vi "S2DS_DetermineTargetInX.vi"(2 "Measurement ON?":bool, 3 "Scan parameters  in":T1 {"Y data taking" items=["in both direction", "in up direction only", "in down direction only"]; "X data taking" items=["in both direction", "in up direction only", "in down direction only"]}) -> (0 "Change  x direction":bool, 1 "Scan parameters  out":T1 {"Y data taking" items=["in both direction", "in up direction only", "in down direction only"]; "X data taking" items=["in both direction", "in up direction only", "in down direction only"]})   [LabVIEW 2025]
uses:
  TYPE DEFS/S2DS_Sweep Info.ctl
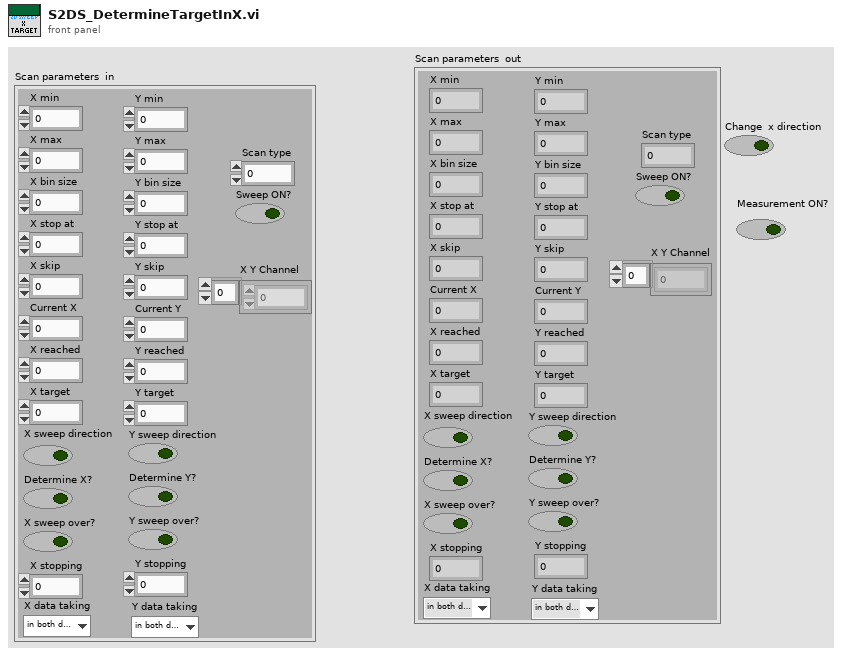
[diagram p1: front panel]
types:
  T1 = typedef "S2DS_Sweep Info.ctl" = cluster{"X min":ext, "X max":dbl, "Y min":dbl, "Y max":dbl, "X bin size":dbl, "Y bin size":dbl, "X stop at":dbl, "Y stop at":dbl, "X skip":u64, "Y skip":u64, "Current X":dbl, "Current Y":dbl, "X reached":i32, "Y reached":i32, "X target":dbl, "Y target":dbl, "Sweep ON?":bool, "X sweep direction":bool, "Y sweep direction":bool, "Determine X?":bool, "Determine Y?":bool, "X sweep over?":bool, "Y sweep over?":bool, "Scan type":i32, "X stopping":i32, "Y stopping":i32, "X Y Channel":u16[], "X data taking":u16, "Y data taking":u16}
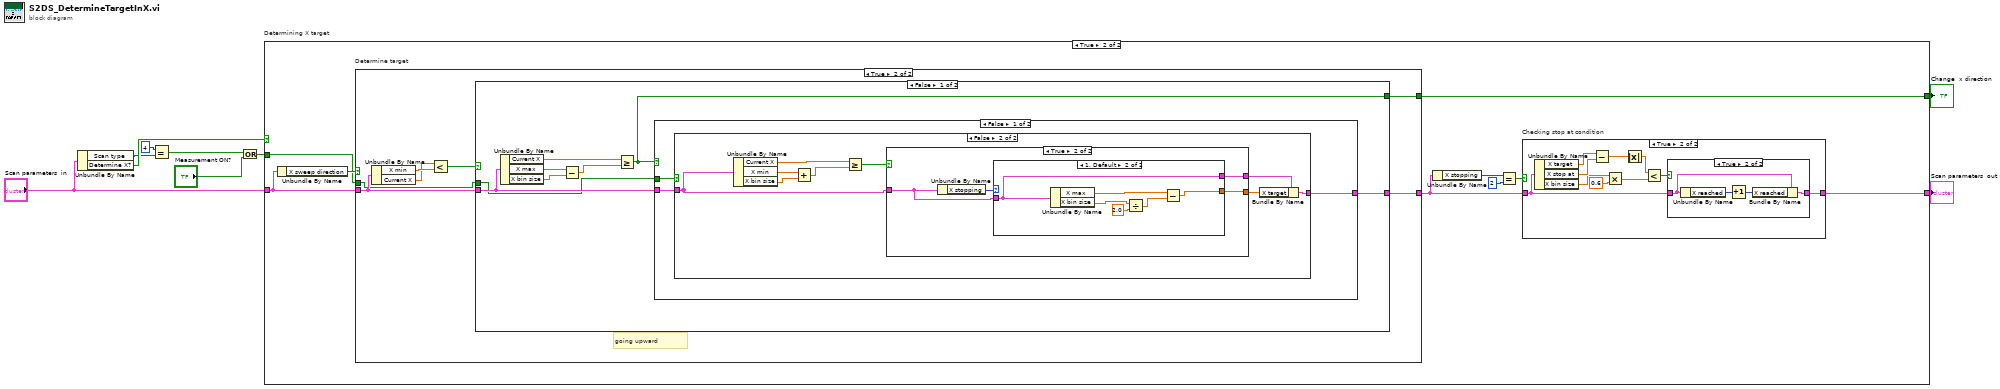
[diagram p0: block diagram]
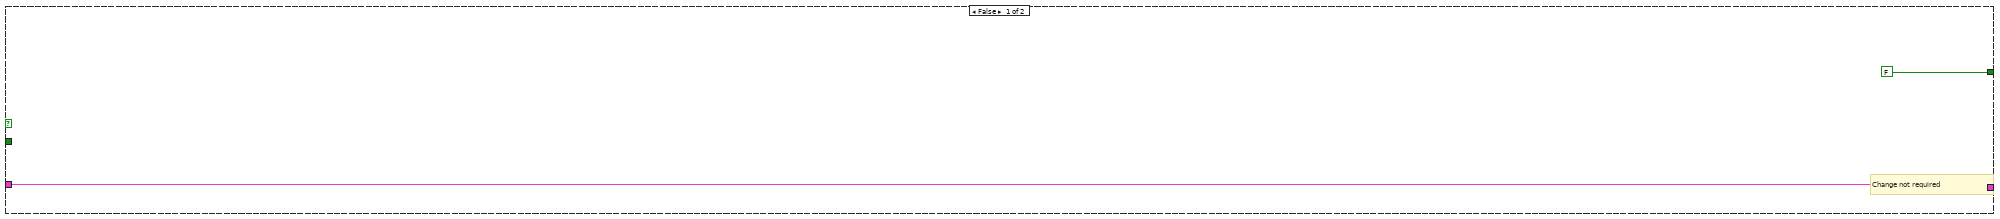
[diagram p2: hidden frame]
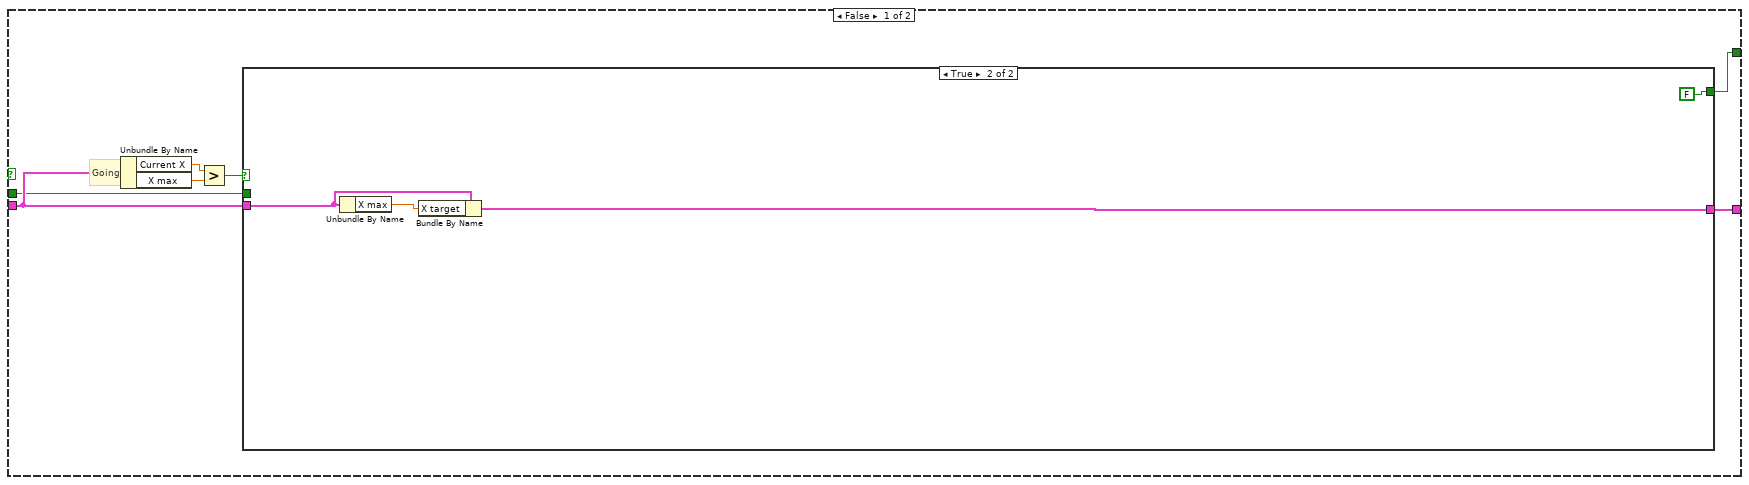
[diagram p3: hidden frame]
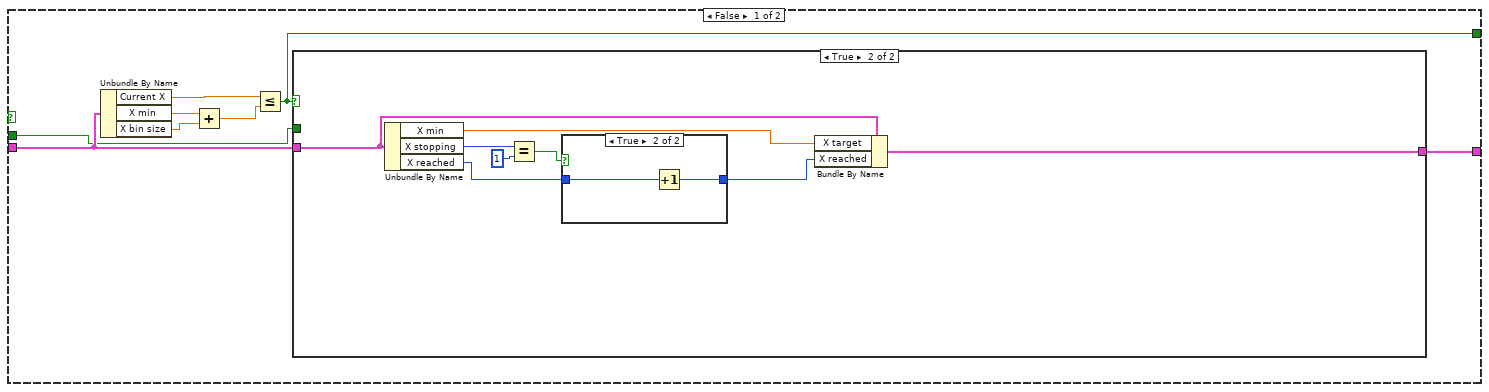
[diagram p4: hidden frame]
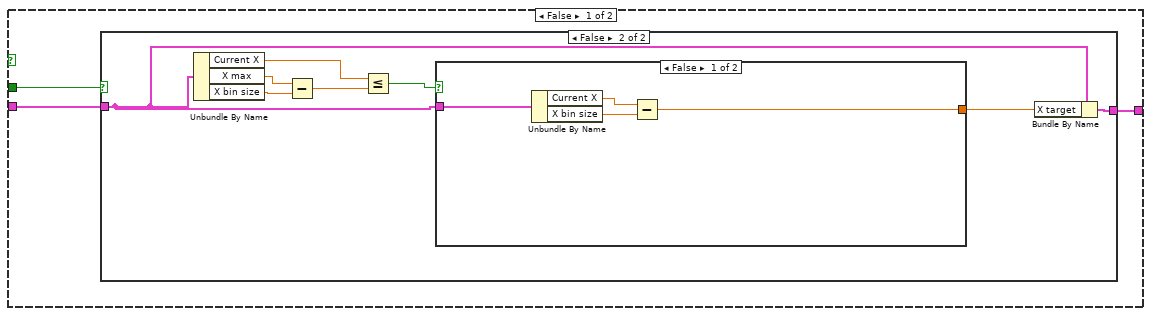
[diagram p5: hidden frame]
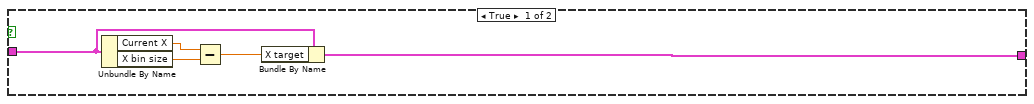
[diagram p6: hidden frame]
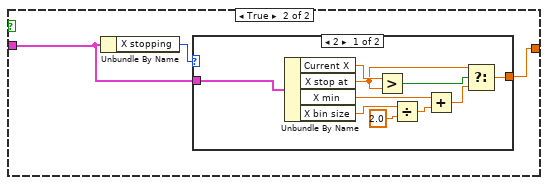
[diagram p7: hidden frame]
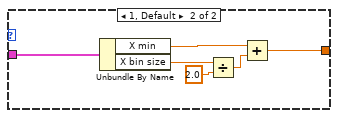
[diagram p8: hidden frame]
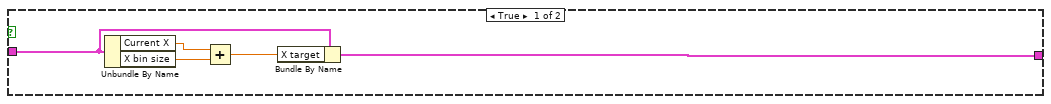
[diagram p10: hidden frame]
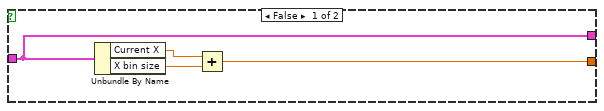
[diagram p11: hidden frame]
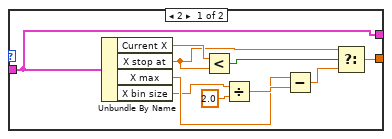
[diagram p12: hidden frame]
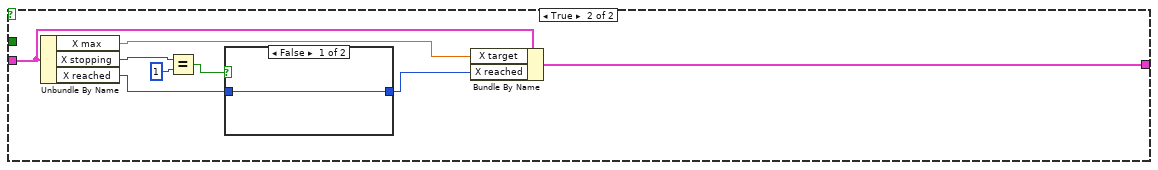
[diagram p13: hidden frame]
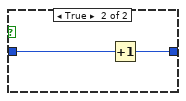
[diagram p14: hidden frame]
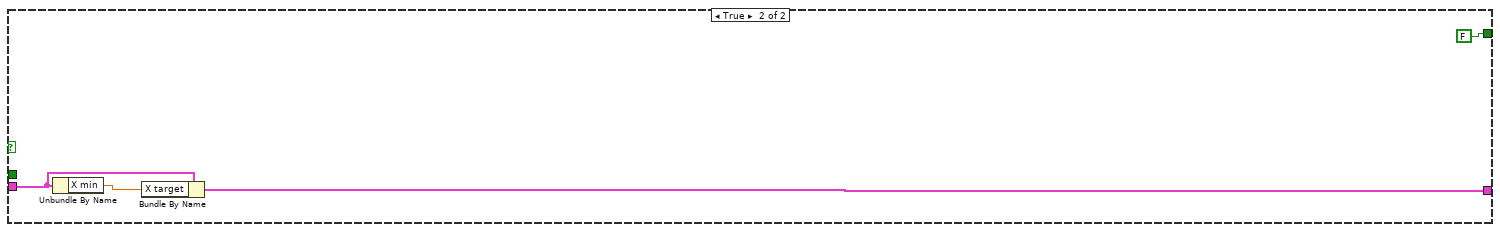
[diagram p15: hidden frame]
diagram:
  n1 = Unbundle By Name("Scan parameters  in") -> ("Scan type"=w5:i32, "Determine X?"=w7:bool)
  n2 = Equal?(x=4, y=w5) -> (x = y?=w3:bool)
  n3 = Or(x=w3, y="Measurement ON?") -> (x .or. y?=w1:bool)
  n4 = case "Determining X target" shown="True" w7 {
    tunnel: "Scan parameters  in" -> [w11 w20]
    tunnel: [w11 w14] -> w9
    tunnel: [FALSE w13] -> w6
    tunnel: w1 -> [_ w12]
    frame False {
      # "Change not required"
    }
    frame True {
      n5 = Unbundle By Name(w20) -> ("X sweep direction"=w18:bool)
      n6 = case "Determine target" shown="True" w18 {
        tunnel: w20 -> [w27 w93]
        tunnel: [w26 w92] -> w19
        tunnel: [w22 w91] -> w13
        tunnel: w12 -> [w21 w90]
        frame False {
          # "Going down"
          n7 = Unbundle By Name(w27) -> ("Current X"=w25:dbl, "X max"=w24:dbl)
          n8 = Greater?(x=w25, y=w24) -> (0:w23:bool)
          n9 = case shown="True" w23 {
            tunnel: w27 -> [w31 w89]
            tunnel: [w30 w87] -> w26
            tunnel: [w29 FALSE] -> w22
            tunnel: w21 -> [w28 _]
            frame False {
              n10 = Unbundle By Name(w31) -> ("Current X"=w33:dbl, "X min"=w35:ext, "X bin size"=w34:dbl)
              n11 = Add(x=w35, y=w34) -> (x+y=w32:ext)
              n12 = Less Or Equal?(x=w33, y=w32) -> (x <= y?=w29:bool)
              n13 = case shown="True" w29 {
                tunnel: w31 -> [w38 w82]
                tunnel: [w37 w80] -> w30
                tunnel: w28 -> [w36 _]
                frame False {
                  n14 = case shown="False" w36 {
                    tunnel: w38 -> [w43 w49]
                    tunnel: [w42 w51] -> w37
                    frame True {
                      n15 = Unbundle By Name(w43) -> ("Current X"=w41:dbl, "X bin size"=w40:dbl)
                      n16 = Subtract(x=w41, y=w40) -> (x-y=w39:dbl)
                      n17 = Bundle By Name(cluster=w43, "X target"=w39) -> (w42:T1)
                    }
                    frame False {
                      n18 = Unbundle By Name(w49) -> ("Current X"=w46:dbl, "X max"=w48:dbl, "X bin size"=w47:dbl)
                      n19 = Subtract(x=w48, y=w47) -> (x-y=w45:dbl)
                      n20 = Less Or Equal?(x=w46, y=w45) -> (x <= y?=w44:bool)
                      n21 = case shown="False" w44 {
                        tunnel: [w52 w58] -> w50
                        tunnel: w49 -> [w53 w57]
                        frame False {
                          n22 = Unbundle By Name(w53) -> ("Current X"=w55:dbl, "X bin size"=w54:dbl)
                          n23 = Subtract(x=w55, y=w54) -> (x-y=w52:dbl)
                        }
                        frame True {
                          n24 = Unbundle By Name(w57) -> ("X stopping"=w56:i32)
                          n25 = case shown="2" w56 {
                            tunnel: w57 -> [w68 w74]
                            tunnel: [w64 w72] -> w58
                            frame 2 {
                              n26 = Unbundle By Name(w68) -> ("Current X"=w67:dbl, "X stop at"=w65:dbl, "X min"=w63:ext, "X bin size"=w62:dbl)
                              n27 = Greater?(x=w67, y=w65) -> (0:w66:bool)
                              n28 = Divide(x=w62, y=2.0) -> (x/y=w60:dbl)
                              n29 = Add(x=w63, y=w60) -> (x+y=w59:ext)
                              n30 = Select(t=w65, s=w66, f=w59) -> (s? t:f=w64:ext)
                            }
                            frame 1, Default {
                              n31 = Unbundle By Name(w74) -> ("X min"=w73:ext, "X bin size"=w71:dbl)
                              n32 = Divide(x=w71, y=2.0) -> (x/y=w69:dbl)
                              n33 = Add(x=w73, y=w69) -> (x+y=w72:ext)
                            }
                          }
                        }
                      }
                      n34 = Bundle By Name(cluster=w49, "X target"=w50) -> (w51:T1)
                    }
                  }
                }
                frame True {
                  n35 = Unbundle By Name(w82) -> ("X min"=w81:ext, "X stopping"=w75:i32, "X reached"=w79:i32)
                  n36 = Equal?(x=w75, y=1) -> (x = y?=w76:bool)
                  n37 = case shown="True" w76 {
                    tunnel: w79 -> [w83 w85]
                    tunnel: [w83 w84] -> w78
                    frame False {
                    }
                    frame True {
                      n38 = Increment(x=w85) -> (x+1=w84:i32)
                    }
                  }
                  n39 = Bundle By Name(cluster=w82, "X target"=w81, "X reached"=w78) -> (w80:T1)
                }
              }
            }
            frame True {
              n40 = Unbundle By Name(w89) -> ("X max"=w88:dbl)
              n41 = Bundle By Name(cluster=w89, "X target"=w88) -> (w87:T1)
            }
          }
        }
        frame True {
          # "going upward"
          n42 = Unbundle By Name(w93) -> ("X min"=w96:ext, "Current X"=w95:dbl)
          n43 = Less?(x=w95, y=w96) -> (x < y?=w94:bool)
          n44 = case shown="False" w94 {
            tunnel: w93 -> [w100 w160]
            tunnel: [w99 w158] -> w92
            tunnel: [w98 FALSE] -> w91
            tunnel: w90 -> [w97 _]
            frame False {
              n45 = Unbundle By Name(w100) -> ("Current X"=w102:dbl, "X max"=w104:dbl, "X bin size"=w103:dbl)
              n46 = Subtract(x=w104, y=w103) -> (x-y=w101:dbl)
              n47 = Greater Or Equal?(x=w102, y=w101) -> (x >= y?=w98:bool)
              n48 = case shown="False" w98 {
                tunnel: w100 -> [w107 w153]
                tunnel: [w106 w151] -> w99
                tunnel: w97 -> [w105 _]
                frame False {
                  n49 = case shown="False" w105 {
                    tunnel: w107 -> [w112 w118]
                    tunnel: [w111 w120] -> w106
                    frame True {
                      n50 = Unbundle By Name(w112) -> ("Current X"=w110:dbl, "X bin size"=w109:dbl)
                      n51 = Add(x=w110, y=w109) -> (x+y=w108:dbl)
                      n52 = Bundle By Name(cluster=w112, "X target"=w108) -> (w111:T1)
                    }
                    frame False {
                      n53 = Unbundle By Name(w118) -> ("Current X"=w115:dbl, "X min"=w117:ext, "X bin size"=w116:dbl)
                      n54 = Add(x=w117, y=w116) -> (x+y=w114:ext)
                      n55 = Greater Or Equal?(x=w115, y=w114) -> (x >= y?=w113:bool)
                      n56 = case shown="True" w113 {
                        tunnel: w118 -> [w122 w129]
                        tunnel: [w122 w127] -> w121
                        tunnel: [w123 w126] -> w119
                        frame False {
                          n57 = Unbundle By Name(w122) -> ("Current X"=w125:dbl, "X bin size"=w124:dbl)
                          n58 = Add(x=w125, y=w124) -> (x+y=w123:dbl)
                        }
                        frame True {
                          n59 = Unbundle By Name(w129) -> ("X stopping"=w128:i32)
                          n60 = case shown="1, Default" w128 {
                            tunnel: w129 -> [w131 w141]
                            tunnel: [w131 w141] -> w127
                            tunnel: [w132 w140] -> w126
                            frame 2 {
                              n61 = Unbundle By Name(w131) -> ("Current X"=w138:dbl, "X stop at"=w130:dbl, "X max"=w135:dbl, "X bin size"=w134:dbl)
                              n62 = Less?(x=w138, y=w130) -> (x < y?=w139:bool)
                              n63 = Divide(x=w134, y=2.0) -> (x/y=w136:dbl)
                              n64 = Subtract(x=w135, y=w136) -> (x-y=w133:dbl)
                              n65 = Select(t=w130, s=w139, f=w133) -> (s? t:f=w132:dbl)
                            }
                            frame 1, Default {
                              n66 = Unbundle By Name(w141) -> ("X max"=w145:dbl, "X bin size"=w144:dbl)
                              n67 = Divide(x=w144, y=2.0) -> (x/y=w142:dbl)
                              n68 = Subtract(x=w145, y=w142) -> (x-y=w140:dbl)
                            }
                          }
                        }
                      }
                      n69 = Bundle By Name(cluster=w121, "X target"=w119) -> (w120:T1)
                    }
                  }
                }
                frame True {
                  n70 = Unbundle By Name(w153) -> ("X max"=w152:dbl, "X stopping"=w146:i32, "X reached"=w150:i32)
                  n71 = Equal?(x=w146, y=1) -> (x = y?=w147:bool)
                  n72 = case shown="False" w147 {
                    tunnel: w150 -> [w154 w156]
                    tunnel: [w154 w155] -> w149
                    frame False {
                    }
                    frame True {
                      n73 = Increment(x=w156) -> (x+1=w155:i32)
                    }
                  }
                  n74 = Bundle By Name(cluster=w153, "X target"=w152, "X reached"=w149) -> (w151:T1)
                }
              }
            }
            frame True {
              n75 = Unbundle By Name(w160) -> ("X min"=w159:ext)
              n76 = Bundle By Name(cluster=w160, "X target"=w159) -> (w158:T1)
            }
          }
        }
      }
      n77 = Unbundle By Name(w19) -> ("X stopping"=w16:i32)
      n78 = Equal?(x=w16, y=2) -> (x = y?=w15:bool)
      n79 = case "Checking stop at condition" shown="True" w15 {
        tunnel: w19 -> [w161 w163]
        tunnel: [w161 w162] -> w14
        frame False {
        }
        frame True {
          n80 = Unbundle By Name(w163) -> ("X target"=w171:dbl, "X stop at"=w170:dbl, "X bin size"=w167:dbl)
          n81 = Subtract(x=w171, y=w170) -> (x-y=w169:dbl)
          n82 = Multiply(x=w167, y=0.6) -> (x*y=w165:dbl)
          n83 = Absolute Value(x=w169) -> (abs(x)=w166:dbl)
          n84 = Less?(x=w166, y=w165) -> (x < y?=w164:bool)
          n85 = case shown="True" w164 {
            tunnel: w163 -> [w172 w175]
            tunnel: [w172 w174] -> w162
            frame False {
            }
            frame True {
              n86 = Unbundle By Name(w175) -> ("X reached"=w176:i32)
              n87 = Increment(x=w176) -> (x+1=w173:i32)
              n88 = Bundle By Name(cluster=w175, "X reached"=w173) -> (w174:T1)
            }
          }
        }
      }
    }
  }
  "Scan parameters  out" <- w9
  "Change  x direction" <- w6
